vi "CANFrame Duration.vi"(8 "error in (no error)":errorcluster, 10 "CAN frame":T1 {"payload" format="%x"; "timestamp" format="%<%.7X\n%x>T"; "type" items=["CAN Data"=0, "CAN Remote"=1, "CAN Bus Error"=2, "CAN 2.0 Data"=8, "CAN FD Data"=16, "CAN FD+BRS Data"=24, "J1939 Data"=192, "Delay"=224, "Log Trigger"=225, "Start Trigger"=226]; "identifier" format="%x"}, 11 "CANBus_Load_Calculator in":refnum<class "CANBus_Load_Calculator.lvclass">) -> (0 "error out":errorcluster, 2 "Frame Duration (us)":u64, 3 "CANBus_Load_Calculator out":refnum<class "CANBus_Load_Calculator.lvclass">)   [LabVIEW 2018, in "NI-XNET Monitor Engine.lvlib" / "XNET-Bus-Load-Calculator.lvlib" / "CANBus_Load_Calculator.lvclass"]
uses:
  CANBus_Load_Calculator.lvclass
  <vilib>/xnet/xnet.llb/XNET Frame CAN.ctl
  <vilib>/xnet/xnet.llb/XNET Frame Type CAN.ctl
  CANBus_Load_Calculator.lvclass/CANBus_Load_Calculator.ctl
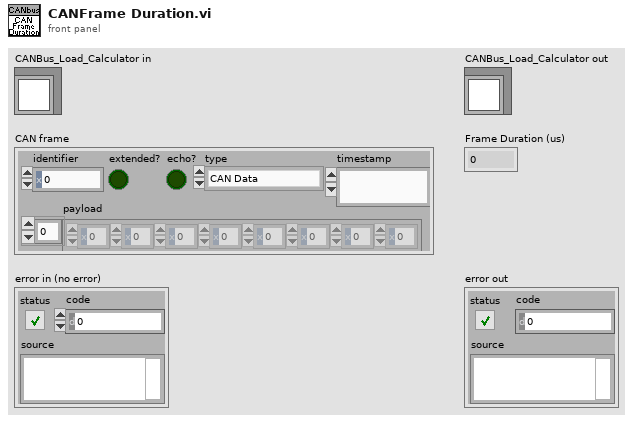
[diagram p1: front panel]
types:
  T1 = typedef "XNET Frame CAN.ctl" = cluster{"timestamp":timestamp, "payload":u8[], "identifier":u32, "type":T2, "extended?":bool, "echo?":bool}
  T2 = typedef "XNET Frame Type CAN.ctl" = u8
  T3 = typedef "NI-XNET Monitor Engine.lvlib/XNET-Bus-Load-Calculator.lvlib/CANBus_Load_Calculator.lvclass/CANFD_Frame_Timing.ctl" = cluster{"Frame Length (Bytes)":i32, "FD.StdID.AvgDuration (us)":u32, "FD.ExtID.AvgDuration (us)":u32, "FDBRS.StdID.AvgDuration (us)":u32, "FDBRS.ExtID.AvgDuration (us)":u32}
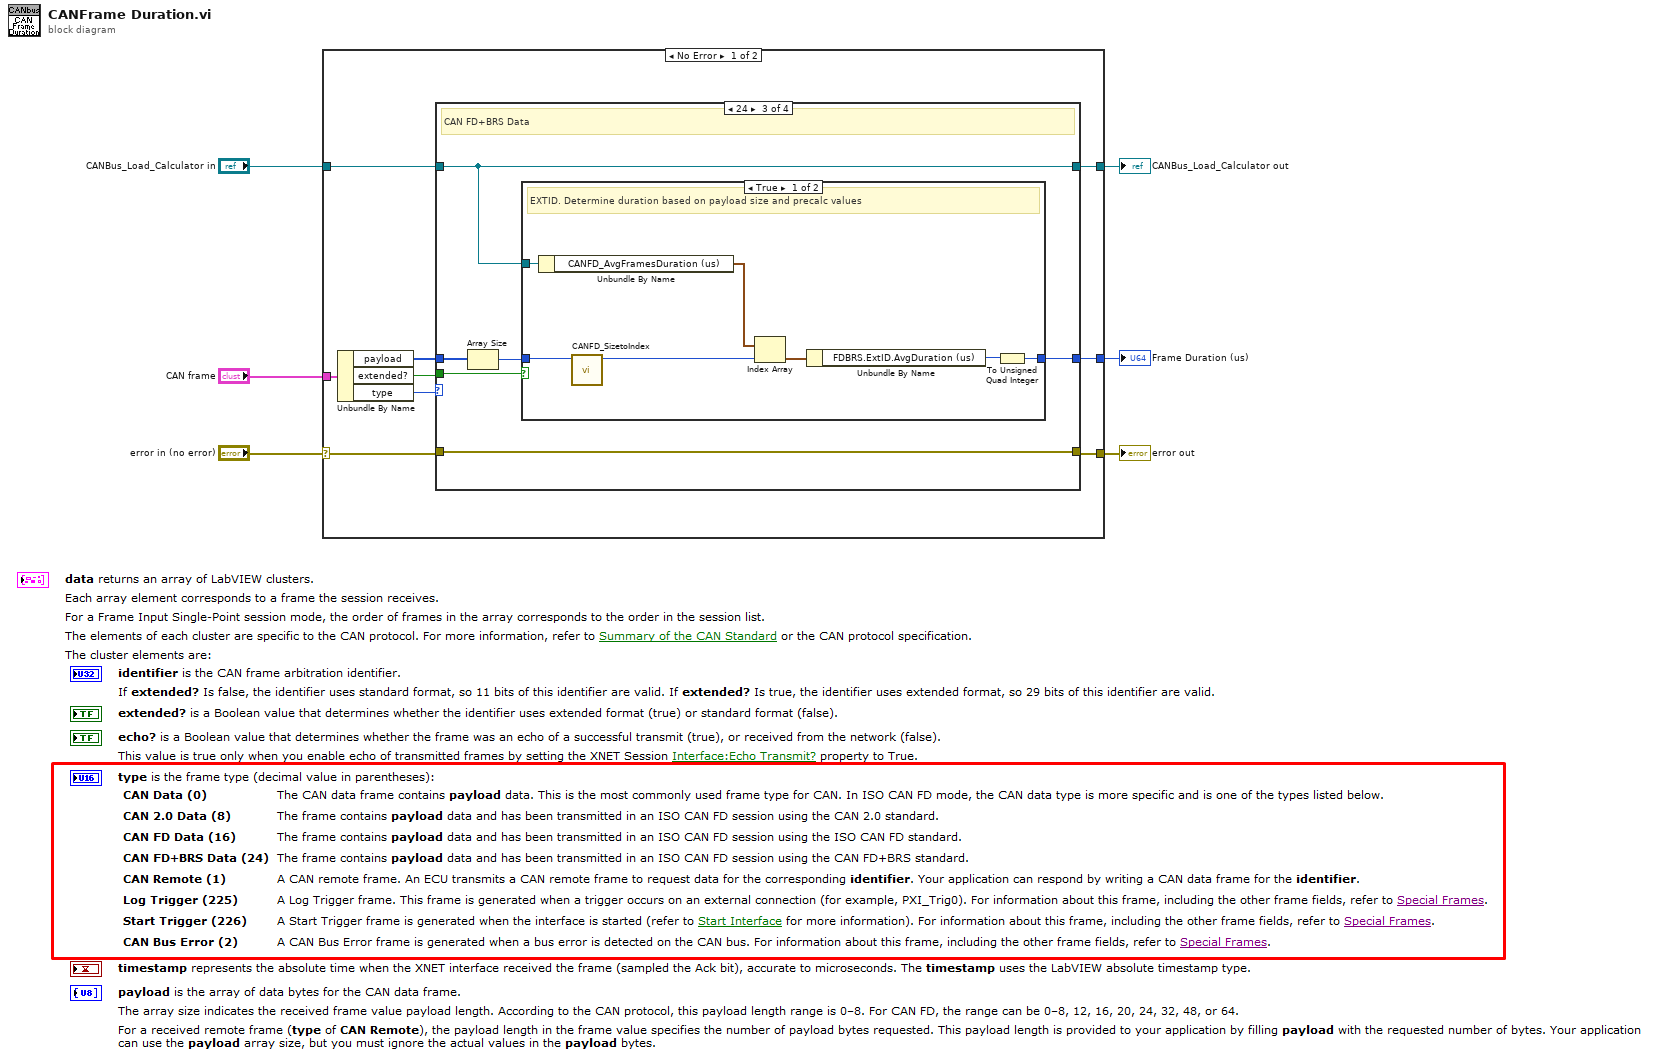
[diagram p0: block diagram]
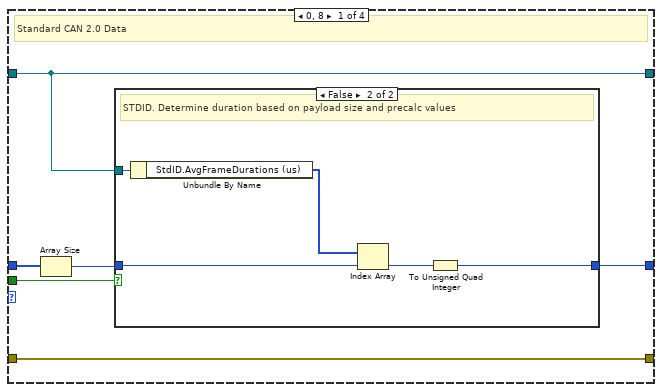
[diagram p2: hidden frame]
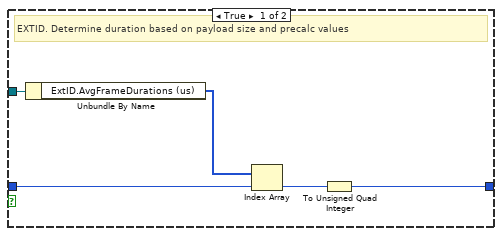
[diagram p3: hidden frame]
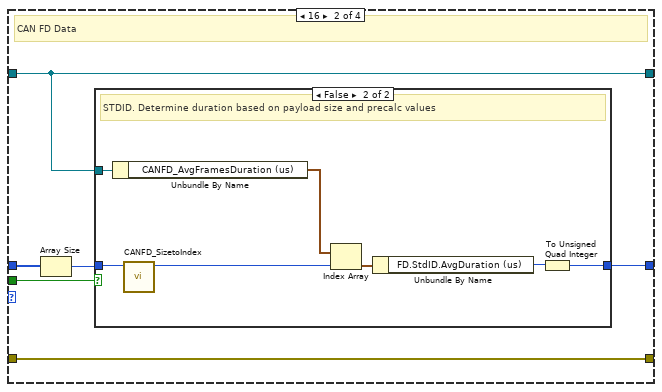
[diagram p4: hidden frame]
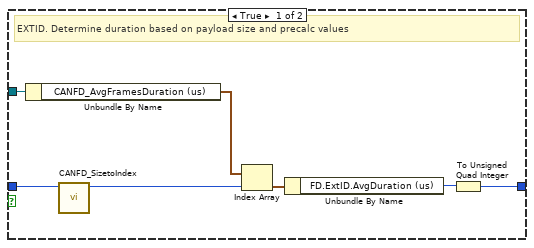
[diagram p5: hidden frame]
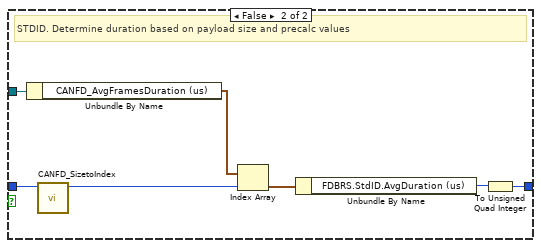
[diagram p6: hidden frame]
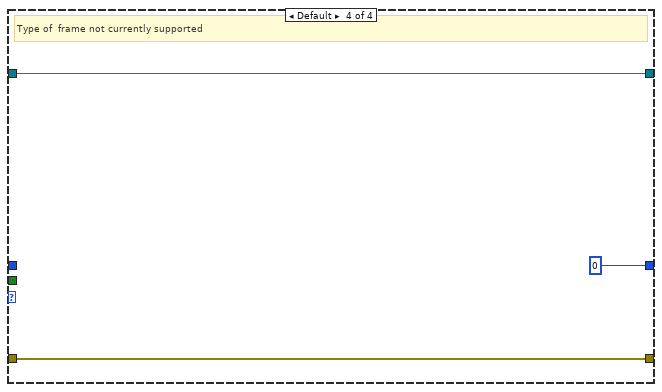
[diagram p7: hidden frame]
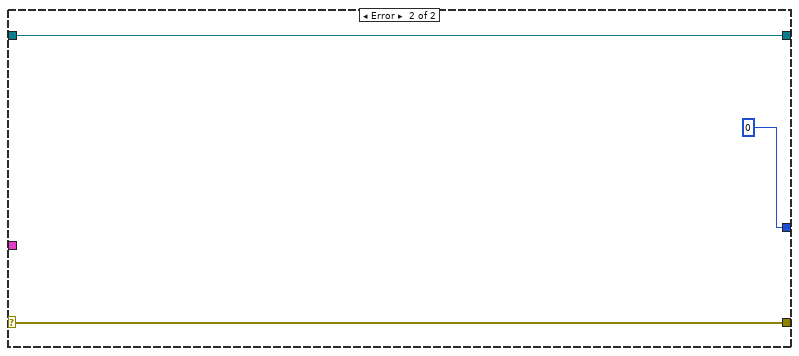
[diagram p8: hidden frame]
diagram:
  n1 = case shown="No Error" "error in (no error)" {
    selector: "error in (no error)" -> [w7 w77]
    tunnel: [w15 u64 0] -> w6
    tunnel: "CANBus_Load_Calculator in" -> [w12 w75]
    tunnel: [w11 w75] -> w4
    tunnel: [w9 w77] -> w3
    tunnel: "CAN frame" -> [w8 _]
    frame No Error {
      n2 = Unbundle By Name(w8) -> ("payload"=w14:u8[], "extended?"=w10:bool, "type"=w13:T2)
      n3 = case shown="24" w13 {
        tunnel: [w21 w37 w57 w74] -> w9
        tunnel: w7 -> [w21 w37 w57 w74]
        tunnel: w10 -> [w20 w36 w56 _]
        tunnel: [w17 w33 w53 w73] -> w11
        tunnel: w12 -> [w17 w33 w53 w73]
        tunnel: w14 -> [w19 w35 w55 _]
        tunnel: [w16 w32 w52 u64 0] -> w15
        frame 0, 8 {
          # "Standard CAN 2.0 Data"
          n4 = Array Size(array=w19) -> (size(s)=w18:i32)
          n5 = case shown="False" w20 {
            tunnel: w18 -> [w24 w29]
            tunnel: w17 -> [w26 w31]
            tunnel: [w22 w27] -> w16
            frame True {
              # "EXTID. Determine duration based on payload size and precalc values"
              n6 = Unbundle By Name(w26) -> ("ExtID.AvgFrameDurations (us)"=w25:u32[])
              n7 = Index Array "Index Array"(array=w25, index=w24) -> (element=w23:u32)
              n8 = To Unsigned Quad Integer(1:w23) -> (0:w22:u64)
            }
            frame False {
              # "STDID. Determine duration based on payload size and precalc values"
              n9 = Unbundle By Name(w31) -> ("StdID.AvgFrameDurations (us)"=w30:u32[])
              n10 = Index Array "Index Array"(array=w30, index=w29) -> (element=w28:u32)
              n11 = To Unsigned Quad Integer(1:w28) -> (0:w27:u64)
            }
          }
        }
        frame 16 {
          # "CAN FD Data"
          n12 = Array Size(array=w35) -> (size(s)=w34:i32)
          n13 = case shown="False" w36 {
            tunnel: w34 -> [w40 w46]
            tunnel: w33 -> [w41 w51]
            tunnel: [w39 w47] -> w32
            frame True {
              # "EXTID. Determine duration based on payload size and precalc values"
              n14 = Unbundle By Name(w41) -> ("CANFD_AvgFramesDuration (us)"=w44:T3[])
              n15 = call "CANFD_SizetoIndex.vi"("Payload Size"=w40) -> ("Duration Index"=w38:i32)  [unwired: 10 in]
              n16 = Index Array "Index Array"(array=w44, index=w38) -> (element=w43:T3)
              n17 = Unbundle By Name(w43) -> ("FD.ExtID.AvgDuration (us)"=w42:u32)
              n18 = To Unsigned Quad Integer(1:w42) -> (0:w39:u64)
            }
            frame False {
              # "STDID. Determine duration based on payload size and precalc values"
              n19 = Unbundle By Name(w51) -> ("CANFD_AvgFramesDuration (us)"=w50:T3[])
              n20 = call "CANFD_SizetoIndex.vi"("Payload Size"=w46) -> ("Duration Index"=w45:i32)  [unwired: 10 in]
              n21 = Index Array "Index Array"(array=w50, index=w45) -> (element=w49:T3)
              n22 = Unbundle By Name(w49) -> ("FD.StdID.AvgDuration (us)"=w48:u32)
              n23 = To Unsigned Quad Integer(1:w48) -> (0:w47:u64)
            }
          }
        }
        frame 24 {
          # "CAN FD+BRS Data"
          n24 = Array Size(array=w55) -> (size(s)=w54:i32)
          n25 = case shown="True" w56 {
            tunnel: w54 -> [w60 w66]
            tunnel: w53 -> [w61 w71]
            tunnel: [w59 w67] -> w52
            frame True {
              # "EXTID. Determine duration based on payload size and precalc values"
              n26 = Unbundle By Name(w61) -> ("CANFD_AvgFramesDuration (us)"=w64:T3[])
              n27 = call "CANFD_SizetoIndex.vi"("Payload Size"=w60) -> ("Duration Index"=w58:i32)  [unwired: 10 in]
              n28 = Index Array "Index Array"(array=w64, index=w58) -> (element=w63:T3)
              n29 = Unbundle By Name(w63) -> ("FDBRS.ExtID.AvgDuration (us)"=w62:u32)
              n30 = To Unsigned Quad Integer(1:w62) -> (0:w59:u64)
            }
            frame False {
              # "STDID. Determine duration based on payload size and precalc values"
              n31 = Unbundle By Name(w71) -> ("CANFD_AvgFramesDuration (us)"=w70:T3[])
              n32 = call "CANFD_SizetoIndex.vi"("Payload Size"=w66) -> ("Duration Index"=w65:i32)  [unwired: 10 in]
              n33 = Index Array "Index Array"(array=w70, index=w65) -> (element=w69:T3)
              n34 = Unbundle By Name(w69) -> ("FDBRS.StdID.AvgDuration (us)"=w68:u32)
              n35 = To Unsigned Quad Integer(1:w68) -> (0:w67:u64)
            }
          }
        }
        frame Default {
          # "Type of  frame not currently supported"
        }
      }
    }
    frame Error {
    }
  }
  "Frame Duration (us)" <- w6
  "CANBus_Load_Calculator out" <- w4
  "error out" <- w3
